vi "LinearSystemLoop_SngJntArm_Execute.vi"(5 "LinearSystem_ID_SngJntArm_Model":T2={"DCMOTOR_TYPES"=enum."NEO", "Num Motors"=1, "ArmLength_M"=0.75, "massKg"=26.0, "Gearing"=128.0, "MOI kgm2"=26.0, "Estimate MOI"=TRUE} {"MOI kgm2" format="%#_13g"; "Gearing" format="%#_13g"; "massKg" format="%#_13g"; "ArmLength_M" format="%#_13g"}, 6 "dT Sec":dbl=0.02, 7 "LinearSystem_SngJntArm_Ctrl_Params":T1={"Ang Model Std Dev Rad"=0.5, "Ang Meas Std Dev Rad"=0.02, "Ang Ctrl Tol Rad"=0.06, "Max Ctrl Out V"=12.0, "Vel Model Std Dev Rad/Sec"=20.0, "Vel Ctrl Tol Rad/Sec"=0.8}, 9 "Process Variable\nRadians":dbl, 10 "Ang Vel SP Rad":dbl format="%#_13g", 11 "Ang Pos SP Rad":dbl) -> (0 "Error":bool, 2 "Filtered Process\nVariable Radians":dbl, 3 "Motor Dmd":dbl, 4 "out Linear System Loop":T4)   [LabVIEW 2019, in "Trajectory_Library.lvlib"]
uses:
  TypeDef/LINEAR_SYSTEM_LOOP.ctl
  TypeDef/LINEAR_QUADRATIC_REGULATOR.ctl
  <vilib>/Analysis/Matrix/Datatypes/RealMatrix.ctl
  TypeDef/LINEAR_PLANT_INV_FF.ctl
  TypeDef/KALMAN_FILTER.ctl
  TypeDef/LINEAR_SYSTEM.ctl
  TypeDef/LINEAR_SYSTEM_ID_SINGLE_JOINT_ARM_MODEL.ctl
  Enum/DCMOTOR_TYPES_ENUM.ctl
  TypeDef/LINEAR_SYSTEM_LOOP_SNGJNTARM_CTRL_PARAMS.ctl
  MatBuilder_Create.vi
  DCMotor_GetCIM.vi
  DCMotor_GetAndymark9015.vi
  DCMotor_GetAndymarkRs775_125.vi
  DCMotor_GetBag.vi
  DCMotor_GetBanebotsRs550.vi
  DCMotor_GetBanebotsRs775.vi
  DCMotor_GetFalcon500.vi
  DCMotor_GetMiniCIM.vi
  DCMotor_GetNEO.vi
  DCMotor_GetNEO550.vi
  DCMotor_GetRomiBuiltIn.vi
  DCMotor_GetVex775Pro.vi
  DCMotor_GetAndymarkAM2235A.vi
  DCMotor_GetAndymarkAM3493.vi
  LinearSystem_New.vi
  MatrixHelper_Zero.vi
  MatBuilder_Fill.vi
  DCMotor_New.vi
  Units_RotationsPerMinuteToRadiansPerSecond.vi
  MatrixHelper_CoerceSize.vi
  Trajectory_Library.lvlib
  <vilib>/Analysis/Matrix/NI_Matrix.lvlib
panel:
  # "<States,1>"
  # "<FUTURE --- CLAMP TYPE -- For now\nuse Normalize>"
  # "Steady State Gain  \n<States,Outputs>"
  # "State Estimate <Statess,1>"
  # "<States,States>"
  # "<States,Inputs>"
  # "<Outputs,States>"
  # "<Outputs,Inputs>"
  # "<States,1>"
  # "<Inputs,1>"
  # "<States,Inputs>"
  # "<States,States>"
  # "Ref State <States,1>"
  # "Comp and capped \noutput <Inputs,1>"
  # "Controller gain\n<Inputs,States>"
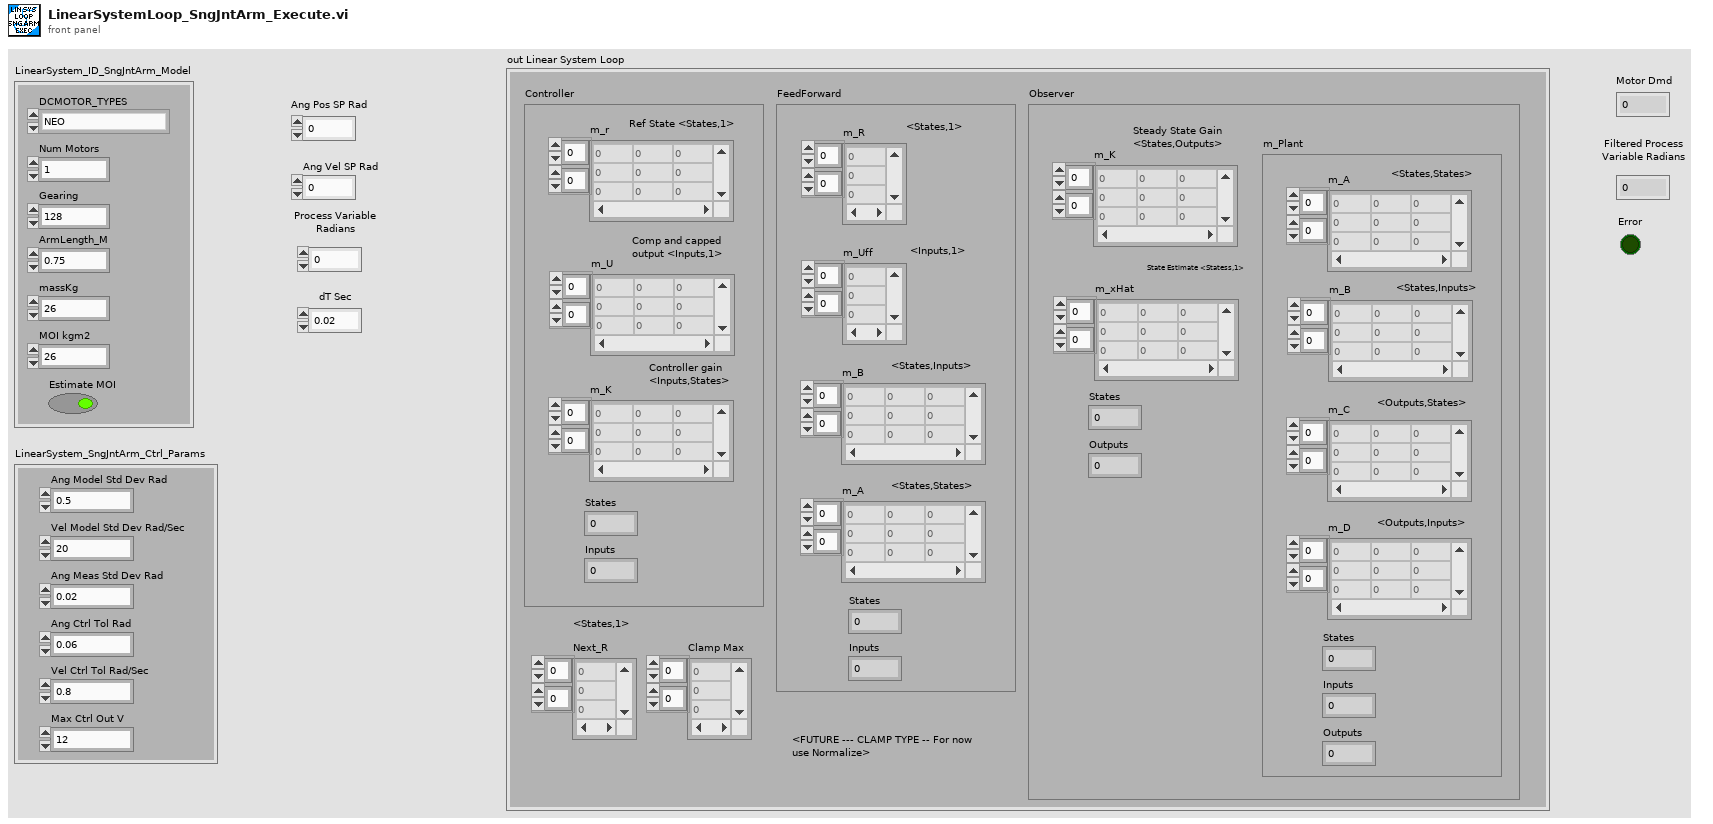
[diagram p1: front panel]
types:
  T1 = typedef "Trajectory_Library.lvlib/LINEAR_SYSTEM_LOOP_SNGJNTARM_CTRL_PARAMS.ctl" = cluster{"Ang Model Std Dev Rad":dbl, "Ang Meas Std Dev Rad":dbl, "Ang Ctrl Tol Rad":dbl, "Max Ctrl Out V":dbl, "Vel Model Std Dev Rad/Sec":dbl, "Vel Ctrl Tol Rad/Sec":dbl}
  T2 = typedef "Trajectory_Library.lvlib/LINEAR_SYSTEM_ID_SINGLE_JOINT_ARM_MODEL.ctl" = cluster{"DCMOTOR_TYPES":T3, "Num Motors":i32, "ArmLength_M":dbl, "massKg":dbl, "Gearing":dbl, "MOI kgm2":dbl, "Estimate MOI":bool}
  T3 = typedef "Trajectory_Library.lvlib/DCMOTOR_TYPES_ENUM.ctl" = enum16{"CIM", "AndyMark 9015", "Andy Mark RS 775 125", "Bag", "BaneBots RS 550", "BaneBots RS 775", "Falcon 500", "Mini CIM", "NEO", "NEO 550", "Romi BuiltIn", "Vex 775 Pro", "Snow Blower AM 2235A", "Bosch Seat AM 3493"}
  T4 = typedef "Trajectory_Library.lvlib/LINEAR_SYSTEM_LOOP.ctl" = cluster{"Controller":T5, "FeedForward":T7, "Observer":T8, "Next_R":T6, "Clamp Max":T6}
  T5 = typedef "Trajectory_Library.lvlib/LINEAR_QUADRATIC_REGULATOR.ctl" = cluster{"m_r":T6, "m_U":T6, "m_K":T6, "States":i32, "Inputs":i32}
  T6 = typedef "NI_Matrix.lvlib/RealMatrix.ctl" = dbl[][]
  T7 = typedef "Trajectory_Library.lvlib/LINEAR_PLANT_INV_FF.ctl" = cluster{"m_R":T6, "m_Uff":T6, "m_B":T6, "m_A":T6, "States":i32, "Inputs":i32}
  T8 = typedef "Trajectory_Library.lvlib/KALMAN_FILTER.ctl" = cluster{"m_K":T6, "m_xHat":T6, "States":i32, "Outputs":i32, "m_Plant":T9}
  T9 = typedef "Trajectory_Library.lvlib/LINEAR_SYSTEM.ctl" = cluster{"m_A":T6, "m_B":T6, "m_C":T6, "m_D":T6, "States":i32, "Inputs":i32, "Outputs":i32}
  T10 = typedef "Trajectory_Library.lvlib/DCMOTOR.CTL" = cluster{"nominalVoltage_Volts":dbl, "StallTorque_NM":dbl, "StallCurrent_Amps":dbl, "FreeCurrent_Amps":dbl, "FreeSpeed_RadPerSec":dbl, "R_Ohms":dbl, "KvINV_RadPerSecPerVolt":dbl, "Kt_NMPerAmp":dbl, "L_H":dbl, "Jr_KgM2":dbl}
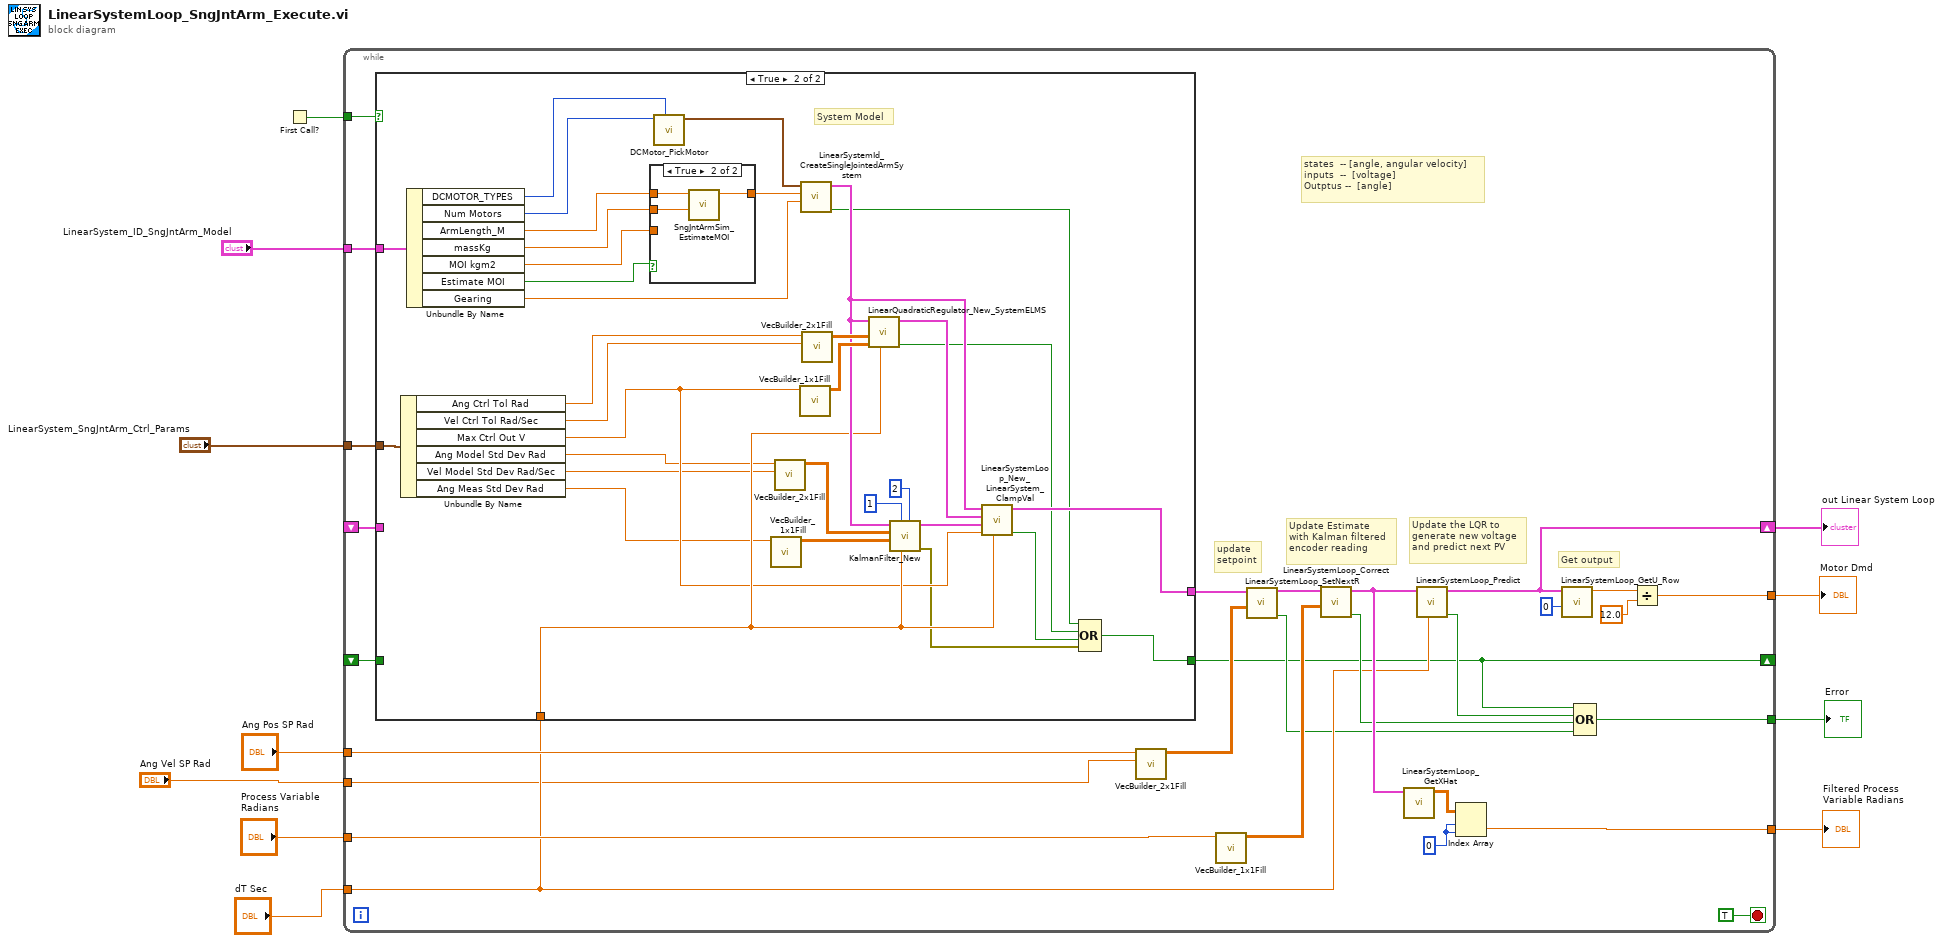
[diagram p0: block diagram]
diagram:
  n1 = First Call?() -> (First Call?: T/F=w3:bool)
  n2 = while {
    tunnel: "Ang Pos SP Rad" -> [w39]
    tunnel: "Process Variable\nRadians" -> [w37]
    tunnel: [w32] -> w8
    tunnel: [w26] -> w7
    tunnel: [w23] -> w6
    tunnel: "dT Sec" -> [w20]
    tunnel: "LinearSystem_ID_SngJntArm_Model" -> [w21]
    shift-right: [w35] -> w9
    shift-left: _ -> [w18]
    tunnel: w3 -> [w17]
    tunnel: "Ang Vel SP Rad" -> [w16]
    tunnel: "LinearSystem_SngJntArm_Ctrl_Params" -> [w15]
    shift-right: [w13] -> _
    shift-left: _ -> [w12]
    stop <- TRUE stop-if-true
    w30 = 0 ("index (row)")
    # "states  -- [angle, angular velocity] \ninputs  --  [voltage]\nOutptus --  [angle]"
    # "Get output"
    # "Update the LQR to \ngenerate new voltage\nand predict next PV"
    # "update \nsetpoint"
    # "Update Estimate\nwith Kalman filtered\nencoder reading"
    n3 = case shown="True" w17 {
      tunnel: w21 -> [_ w72]
      tunnel: w20 -> [_ w54]
      tunnel: [w41 w55] -> w19
      tunnel: w18 -> [w41 _]
      tunnel: w15 -> [_ w53]
      tunnel: [w40 w42] -> w13
      tunnel: w12 -> [w40 _]
      frame False {
      }
      frame True {
        # "System Model"
        n4 = Unbundle By Name(w53) -> ("Ang Ctrl Tol Rad"=w52:dbl, "Vel Ctrl Tol Rad/Sec"=w51:dbl, "Max Ctrl Out V"=w50:dbl, "Ang Model Std Dev Rad"=w49:dbl, "Vel Model Std Dev Rad/Sec"=w48:dbl, "Ang Meas Std Dev Rad"=w47:dbl)
        n5 = Unbundle By Name(w72) -> ("DCMOTOR_TYPES"=w66:T3, "Num Motors"=w65:i32, "ArmLength_M"=w71:dbl, "massKg"=w70:dbl, "MOI kgm2"=w68:dbl, "Estimate MOI"=w69:bool, "Gearing"=w67:dbl)
        n6 = case shown="True" w69 {
          tunnel: [w75 w78] -> w74
          tunnel: w71 -> [_ w77]
          tunnel: w70 -> [_ w76]
          tunnel: w68 -> [w75 _]
          frame False {
          }
          frame True {
            n7 = call "SngJntArmSim_EstimateMOI.vi"("ArmMass_Kg"=w76, "ArmLength_M"=w77) -> ("MOI"=w78:dbl)  [unwired: 9 in]
          }
        }
        n8 = call "DCMotor_PickMotor.vi"("DCMOTOR_TYPES"=w66, "Num Motors"=w65) -> ("DCMOTOR"=w73:T10)  [unwired: 9 in]
        n9 = call "VecBuilder_1x1Fill.vi"("R0_C0"=w47) -> ("output matrix"=w64:T6)  [unwired: 10 in]
        n10 = call "VecBuilder_2x1Fill.vi"("R1"=w48, "R0"=w49) -> ("output matrix"=w63:T6)  [unwired: 9 in]
        n11 = call "VecBuilder_1x1Fill.vi"("R0_C0"=w50) -> ("output matrix"=w61:T6)  [unwired: 10 in]
        n12 = call "LinearSystemId_CreateSingleJointedArmSystem.vi"("G"=w67, "jKgSquaredMeters"=w74, "DCMOTOR"=w73) -> ("Size Coerced"=w46:bool, "Linearsystem"=w59:T9)  [unwired: 7 in]
        n13 = call "VecBuilder_2x1Fill.vi"("R1"=w51, "R0"=w52) -> ("output matrix"=w60:T6)  [unwired: 9 in]
        n14 = call "LinearQuadraticRegulator_New_SystemELMS.vi"("dt_Seconds"=w54, "Relms"=w61, "Qelms"=w60, "LINEARSYSTEM"=w59) -> ("Error"=w45:bool, "LinearQuadraticRegulator"=w58:T5)  [unwired: 6 in]
        n15 = call "KalmanFilter_New.vi"("States"=2, "dt_Seconds"=w54, "Outputs"=1, "MeasurementStdDevs"=w64, "StateStdDevs"=w63, "Plant"=w59) -> ("Error"=w43:errorcluster, "KalmanFilter"=w56:T8)  [unwired: 4 in]
        n16 = call "LinearSystemLoop_New_LinearSystem_ClampVal.vi"("dT_Seconds"=w54, "Max_Voltage"=w50, "Observer"=w56, "Controller"=w58, "Plant"=w59) -> ("Error"=w44:bool, "Linear System Loop"=w55:T4)  [unwired: 5 in]
        n17 = Compound Arithmetic op=OR(w46, w45, w44, w43) -> (w42:bool)
      }
    }
    n18 = call "VecBuilder_2x1Fill.vi"("R1"=w16, "R0"=w39) -> ("output matrix"=w38:T6)  [unwired: 9 in]
    n19 = call "VecBuilder_1x1Fill.vi"("R0_C0"=w37) -> ("output matrix"=w29:T6)  [unwired: 10 in]
    n20 = call "LinearSystemLoop_SetNextR.vi"("R"=w38, "input inear System Loop"=w19) -> ("Size Coerced"=w14:bool, "out Linear System Loop"=w36:T4)  [unwired: 8 in]
    n21 = call "LinearSystemLoop_Correct.vi"("Y"=w29, "input inear System Loop"=w36) -> ("Error"=w27:bool, "out Linear System Loop"=w33:T4)  [unwired: 8 in]
    n22 = call "LinearSystemLoop_GetXHat.vi"("input inear System Loop"=w33) -> ("XHat"=w31:T6)  [unwired: 10 in]
    n23 = call "LinearSystemLoop_Predict.vi"("dT_Seconds"=w20, "input inear System Loop"=w33) -> ("Error"=w28:bool, "out Linear System Loop"=w35:T4)  [unwired: 8 in]
    n24 = Index Array(array=w31, index (row)=w30, index (col)=w30) -> (element=w32:dbl)
    n25 = call "LinearSystemLoop_GetU_Row.vi"("Row"=0, "input inear System Loop"=w35) -> ("U"=w25:dbl)  [unwired: 9 in]
    n26 = Compound Arithmetic op=OR(w13, w28, w27, w14) -> (w26:bool)
    n27 = Divide(x=w25, y=12.0) -> (x/y=w23:dbl)
  }
  "Motor Dmd" <- w6
  "out Linear System Loop" <- w9
  "Filtered Process\nVariable Radians" <- w8
  "Error" <- w7
